vi "Is Connected.vi"(6 "Synchronization":enum16{"Start", "Wait"}(ring), 7 "Description":string, 8 "Command Info In":T1) -> (0 "Command Info Out":T1)   [LabVIEW 2018]
doc: "This template has a parameter to control whether it waits for the command to complete or not. This is useful for operations that have a timed duration or a sensor-based duration. \n\nBe sure to right-click and select New from Template and save with a new command name."
uses:
  <vilib>/Rock Robotics/WPI/Framework/Command Status Info.ctl
  <vilib>/Rock Robotics/WPI/Framework/Completion Status.ctl
  <vilib>/Rock Robotics/WPI/Framework/Completion Notifier.ctl
  Implementation/LattePanda Setpoints.ctl
  Implementation/LattePanda Operations.ctl
panel:
  out "Connected?":bool
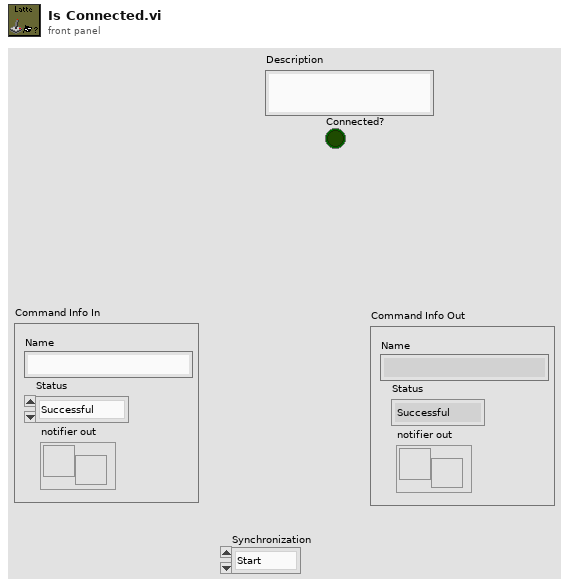
[diagram p1: front panel]
types:
  T1 = typedef "Command Status Info.ctl" = cluster{"Name":string, "Status":T2, "notifier out":T3}
  T2 = typedef "Completion Status.ctl" = enum16{"Successful", "Aborted", "Incomplete"}
  T3 = typedef "Completion Notifier.ctl" = refnum<notifier>
  T4 = typedef "LattePanda Setpoints.ctl" = cluster{"Operation":T5, "Setpoint":dbl, "Duration":dbl, "Connected?":bool}
  T5 = typedef "LattePanda Operations.ctl" = enum16{"Reserve", "Read Current", "Immediate", "Power On", "Shut Down", "Is Conneced"}
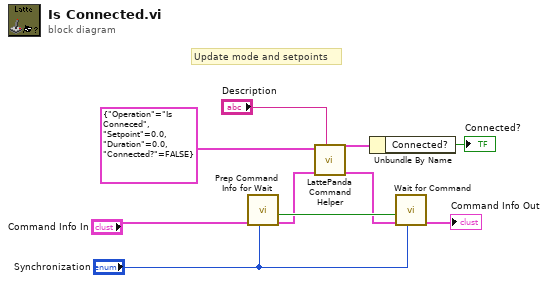
[diagram p0: block diagram]
diagram:
  # "Update mode and setpoints"
  n1 = call <vilib>:"Prep Command Info for Wait.vi"("Synchronication"="Synchronization", "Command Info"="Command Info In") -> ("Command Info"=w8:T1, "Allocated"=w9:bool)  [unwired: 8 in]
  n2 = call "LattePanda Command Helper.vi"("Description"="Description", "Command Info In"=w8, "SubSystem Data"=T4 {"Operation"=enum."Is Conneced", "Setpoint"=0.0, "Duration"=0.0, "Connected?"=FALSE}) -> ("Command Info Out"=w5:T1, "SubSystem Data"=w2:T4)  [unwired: 6 in, 1 out]
  n3 = Unbundle By Name(w2) -> ("Connected?"=→"Connected?":bool)
  n4 = call <vilib>:"Wait for Command.vi"("Synchronication"="Synchronization", "Command Info in"=w5, "Allocated"=w9) -> ("Command Info out"=→"Command Info Out":T1)  [unwired: 8 in]
